vi "DRAM FIFO Pattern Generator.vi"(8 "Generate Point":bool, 11 "Points to Generate":u32) -> (0 "Output Valid":bool, 1 "Generation Done?":bool, 2 "Points Done":u32, 3 "Output Data":T1)   [LabVIEW 2011]
uses:
  Data Type (256).ctl
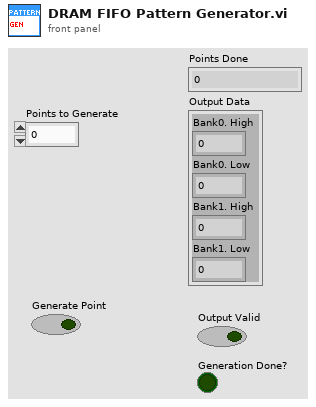
[diagram p1: front panel]
types:
  T1 = typedef "Data Type (256).ctl" = cluster{"Bank0. High":u64, "Bank0. Low":u64, "Bank1. High":u64, "Bank1. Low":u64}
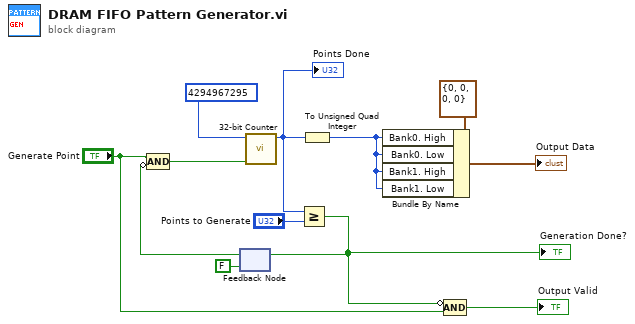
[diagram p0: block diagram]
diagram:
  n1 = feedback #1(FALSE) -> (w6:bool)
  n2 = Compound Arithmetic op=AND("Generate Point", invert w6) -> (w4:bool)
  n3 = call "32-bit Counter.vi"("INC?"=w4, "rollover"=u32 4294967295) -> ("count"=w8:u32)  [unwired: 9 in]
  "Points Done" <- w8
  n4 = Greater Or Equal?(x=w8, y="Points to Generate") -> (x >= y?=w3:bool)
  "Generation Done?" <- w3
  n5 = feedback-in #1(w3) -> ()
  n6 = To Unsigned Quad Integer(1:w8) -> (0:w9:u64)
  n7 = Bundle By Name(cluster=T1 {"Bank0. High"=0, "Bank0. Low"=0, "Bank1. High"=0, "Bank1. Low"=0} ("Input Data"), "Bank0. High"=w9, "Bank0. Low"=w9, "Bank1. High"=w9, "Bank1. Low"=w9) -> (→"Output Data":T1)
  n8 = Compound Arithmetic op=AND(invert w3, "Generate Point") -> (→"Output Valid":bool)
